vi "CAL-Daten laden.vi"(11 "Aktion":enum16{"PMA", "FID"}(ring)) -> (1 "CAL-Daten Tolernaz":T2, 2 "CAL-Daten FID":T1={"CH4 Null"=0.0, "CH4 Steil"=[1.0, 1.0, 1.0, 1.0], "THC Null"=0.0, "THC Steil"=[1.0, 1.0, 1.0, 1.0], "NMHC Null"=0.0, "NMHC Steil"=[1.0, 1.0, 1.0, 1.0]}, 3 "CAL-Daten":T3={"O2 Null"=0.0, "O2 Steil"=[1.0, 1.0, 1.0, 1.0]}, 4 "Aktiv":bool[](array[boolean]), 5 "Polynom":sgl[][](array[numeric]))   [LabVIEW 2020, in "ABB-EL3000.lvlib" / "Allgemeine VI.lvlib"]
uses:
  Allgemeine VI.lvlib
  CAL-Daten PMA.ctl
  CAL-Daten Toleranz.ctl
  CAL-Daten FID.ctl
  <vilib>/Utility/config.llb/Read Key (String).vi
  <vilib>/Utility/config.llb/NI_LVConfig.lvlib
  Allgemein/allgemeine Sub-VIs.lvlib
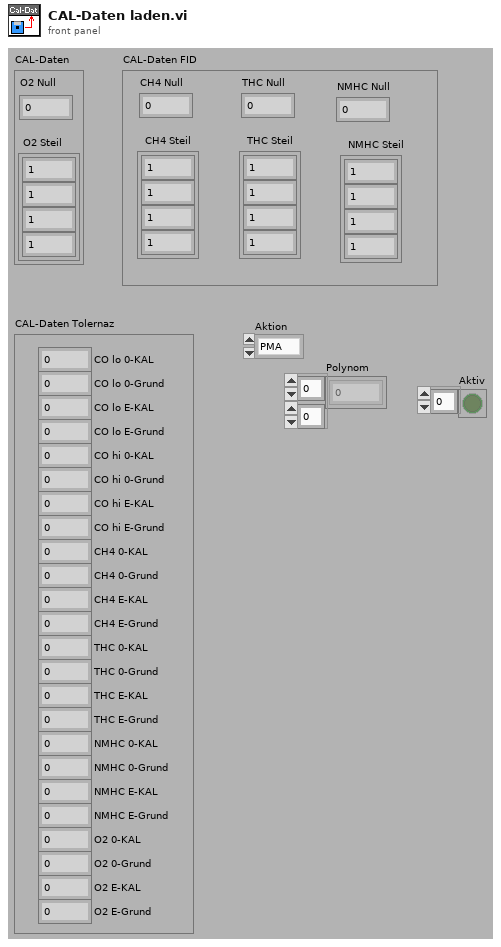
[diagram p1: front panel]
types:
  T1 = typedef "ABB-EL3000.lvlib/Allgemeine VI.lvlib/CAL-Daten FID.ctl" = cluster{"CH4 Null":sgl, "CH4 Steil":sgl[], "THC Null":sgl, "THC Steil":sgl[], "NMHC Null":sgl, "NMHC Steil":sgl[]}
  T2 = typedef "ABB-EL3000.lvlib/Allgemeine VI.lvlib/CAL-Daten Toleranz.ctl" = cluster{"CO lo 0-KAL":sgl, "CO lo 0-Grund":sgl, "CO lo E-KAL":sgl, "CO lo E-Grund":sgl, "CO hi 0-KAL":sgl, "CO hi 0-Grund":sgl, "CO hi E-KAL":sgl, "CO hi E-Grund":sgl, "CH4 0-KAL":sgl, "CH4 0-Grund":sgl, "CH4 E-KAL":sgl, "CH4 E-Grund":sgl, "THC 0-KAL":sgl, "THC 0-Grund":sgl, "THC E-KAL":sgl, "THC E-Grund":sgl, "NMHC 0-KAL":sgl, "NMHC 0-Grund":sgl, "NMHC E-KAL":sgl, "NMHC E-Grund":sgl, "O2 0-KAL":sgl, "O2 0-Grund":sgl, "O2 E-KAL":sgl, "O2 E-Grund":sgl}
  T3 = typedef "ABB-EL3000.lvlib/Allgemeine VI.lvlib/CAL-Daten PMA.ctl" = cluster{"O2 Null":sgl, "O2 Steil":sgl[]}
  T4 = typedef "NI_LVConfig.lvlib/Config Data RefNum.ctl" = refnum<k1>
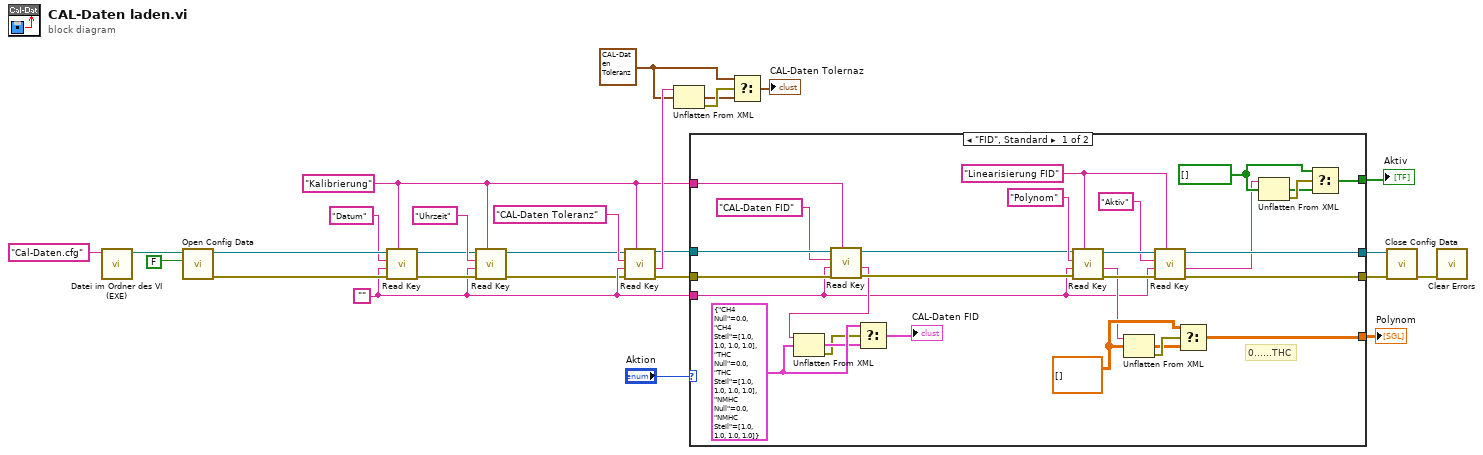
[diagram p0: block diagram]
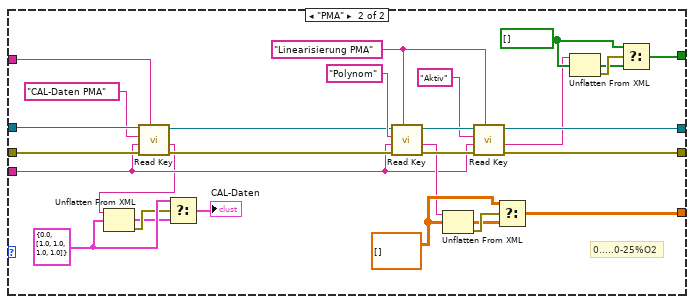
[diagram p2: hidden frame]
diagram:
  w13 = T2 {"CO lo 0-KAL"=2.0, "CO lo 0-Grund"=15.0, "CO lo E-KAL"=2.0, "CO lo E-Grund"=15.0, "CO hi 0-KAL"=2.0, "CO hi 0-Grund"=15.0, "CO hi E-KAL"=2.0, "CO hi E-Grund"=15.0, "CH4 0-KAL"=2.0, "CH4 0-Grund"=15.0, "CH4 E-KAL"=2.0, "CH4 E-Grund"=15.0, "THC 0-KAL"=2.0, "THC 0-Grund"=15.0, "THC E-KAL"=2.0, "THC E-Grund"=15.0, "NMHC 0-KAL"=2.0, "NMHC 0-Grund"=15.0, "NMHC E-KAL"=2.0, "NMHC E-Grund"=15.0, "O2 0-KAL"=0.0, "O2 0-Grund"=0.0, "O2 E-KAL"=0.0, "O2 E-Grund"=0.0} ("CAL-Daten Tolernaz")
  w1 = "Kalibrierung" ("section")
  w9 = ""
  n1 = call "Datei im Ordner des VI (EXE).vi"("Dateiname"="Cal-Daten.cfg") -> ("Dateipfad im Ordner des Haupt-VIs"=w25:path)  [unwired: 8 in, 2 out]
  n2 = call <vilib>:"Open Config Data.vi"("create file if necessary (T)"=FALSE, "configuration file path"=w25) -> ("error out"=w26:errorcluster, "refnum"=w27:T4)  [unwired: 7 in, 1 out]
  n3 = call-poly <vilib>:"Read Key.vi"("section"=w1, "error in (no error)"=w26, "default value"=w9, "key"="Datum", "refnum"=w27) -> ("error out"=w20:errorcluster, "refnum out"=w18:T4)  [unwired: 1 in, 4 out]
  n4 = call-poly <vilib>:"Read Key.vi"("section"=w1, "error in (no error)"=w20, "default value"=w9, "key"="Uhrzeit", "refnum"=w18) -> ("error out"=w2:errorcluster, "refnum out"=w3:T4)  [unwired: 1 in, 4 out]
  n5 = call-poly <vilib>:"Read Key.vi"("section"=w1, "error in (no error)"=w2, "default value"=w9, "key"="CAL-Daten Toleranz", "refnum"=w3) -> ("error out"=w8:errorcluster, "value"=w16:string, "refnum out"=w7:T4)  [unwired: 1 in, 3 out]
  n6 = Unflatten From XML(xml string=w16, type=w13) -> (value=w14:T2, error out=w15:errorcluster)  [unwired: 1 in]
  n7 = case shown="\"FID\", Standard" "Aktion" {
    tunnel: [w54 w83] -> w11
    tunnel: [w53 w82] -> w10
    tunnel: w9 -> [w28 w58]
    tunnel: w8 -> [w38 w68]
    tunnel: w7 -> [w39 w67]
    tunnel: [w41 w70] -> w5
    tunnel: [w40 w69] -> w4
    tunnel: w1 -> [w35 w63]
    frame "FID", Default {
      w32 = T1 {"CH4 Null"=0.0, "CH4 Steil"=[1.0, 1.0, 1.0, 1.0], "THC Null"=0.0, "THC Steil"=[1.0, 1.0, 1.0, 1.0], "NMHC Null"=0.0, "NMHC Steil"=[1.0, 1.0, 1.0, 1.0]} ("CAL-Daten FID")
      w43 = bool[] []
      w47 = sgl[][] []
      w52 = "Linearisierung FID" ("key")
      # "0......THC"
      n8 = call-poly <vilib>:"Read Key.vi"("section"=w35, "error in (no error)"=w38, "default value"=w28, "key"="CAL-Daten FID", "refnum"=w39) -> ("error out"=w36:errorcluster, "value"=w29:string, "refnum out"=w37:T4)  [unwired: 1 in, 3 out]
      n9 = Unflatten From XML(xml string=w29, type=w32) -> (value=w31:T1, error out=w30:errorcluster)  [unwired: 1 in]
      n10 = Select(t=w32, s=w30, f=w31) -> (s? t:f=→"CAL-Daten FID":T1)
      n11 = call-poly <vilib>:"Read Key.vi"("section"=w52, "error in (no error)"=w36, "default value"=w28, "key"="Polynom", "refnum"=w37) -> ("error out"=w55:errorcluster, "value"=w46:string, "refnum out"=w56:T4)  [unwired: 1 in, 3 out]
      n12 = Unflatten From XML(xml string=w46, type=w47) -> (value=w48:sgl[][], error out=w49:errorcluster)  [unwired: 1 in]
      n13 = call-poly <vilib>:"Read Key.vi"("section"=w52, "error in (no error)"=w55, "default value"=w28, "key"="Aktiv", "refnum"=w56) -> ("error out"=w54:errorcluster, "value"=w42:string, "refnum out"=w53:T4)  [unwired: 1 in, 3 out]
      n14 = Select(t=w47, s=w49, f=w48) -> (s? t:f=w41:sgl[][])
      n15 = Unflatten From XML(xml string=w42, type=w43) -> (value=w44:bool[], error out=w45:errorcluster)  [unwired: 1 in]
      n16 = Select(t=w43, s=w45, f=w44) -> (s? t:f=w40:bool[])
    }
    frame "PMA" {
      w62 = T3 {"O2 Null"=0.0, "O2 Steil"=[1.0, 1.0, 1.0, 1.0]} ("CAL-Daten")
      w72 = bool[] []
      w76 = sgl[][] []
      w81 = "Linearisierung PMA" ("key")
      # "0.....0-25%O2"
      n17 = call-poly <vilib>:"Read Key.vi"("section"=w63, "error in (no error)"=w68, "default value"=w58, "key"="CAL-Daten PMA", "refnum"=w67) -> ("error out"=w65:errorcluster, "value"=w57:string, "refnum out"=w66:T4)  [unwired: 1 in, 3 out]
      n18 = Unflatten From XML(xml string=w57, type=w62) -> (value=w60:T3, error out=w61:errorcluster)  [unwired: 1 in]
      n19 = Select(t=w62, s=w61, f=w60) -> (s? t:f=→"CAL-Daten":T3)
      n20 = call-poly <vilib>:"Read Key.vi"("section"=w81, "error in (no error)"=w65, "default value"=w58, "key"="Polynom", "refnum"=w66) -> ("error out"=w84:errorcluster, "value"=w75:string, "refnum out"=w85:T4)  [unwired: 1 in, 3 out]
      n21 = Unflatten From XML(xml string=w75, type=w76) -> (value=w77:sgl[][], error out=w78:errorcluster)  [unwired: 1 in]
      n22 = call-poly <vilib>:"Read Key.vi"("section"=w81, "error in (no error)"=w84, "default value"=w58, "key"="Aktiv", "refnum"=w85) -> ("error out"=w83:errorcluster, "value"=w71:string, "refnum out"=w82:T4)  [unwired: 1 in, 3 out]
      n23 = Select(t=w76, s=w78, f=w77) -> (s? t:f=w70:sgl[][])
      n24 = Unflatten From XML(xml string=w71, type=w72) -> (value=w73:bool[], error out=w74:errorcluster)  [unwired: 1 in]
      n25 = Select(t=w72, s=w74, f=w73) -> (s? t:f=w69:bool[])
    }
  }
  "Polynom" <- w5
  "Aktiv" <- w4
  n26 = Select(t=w13, s=w15, f=w14) -> (s? t:f=→"CAL-Daten Tolernaz":T2)
  n27 = call <vilib>:"Close Config Data.vi"("error in (no error)"=w11, "refnum"=w10) -> ("error out"=w22:errorcluster)  [unwired: 1 in, 8 out]
  n28 = call <vilib>:"Clear Errors.vi"("error in (no error)"=w22) -> ()  [unwired: 5 in, 2 out]
